vi "ATS_AsyncGetSetBufCount.vi"(9 "Get / Set&Get":bool, 10 "BuffCount":i32, 11 "DeviceIn":i32) -> (0 "Return Code":u32, 2 "BufCount_Out":i32, 3 "DeviceOut":i32)   [LabVIEW 2012]
doc: "_____AlazarTech, Scope_____\n\nGet or Set and Get the Buffer Count use in the AsyncDMA mode.\n\nBuffCount_Out is the value already set for the AsyncDMA read."
uses:
  ATS_ctl/ATS_Global_Ctrl.ctl
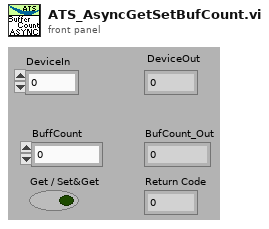
[diagram p1: front panel]
types:
  T1 = typedef "ATS_Global_Ctrl.ctl" = enum16{"Init_Device", "Clear_ALL", "Set", "Get"}
  T2 = typedef "Device_Info.ctl" = cluster{"Handle":u32, "Board":string, "CPLD":string, "MemorySize":u32, "SampleSize":u8, "ID":i32, "High_Memory":bool, "Chan/Board":u8}
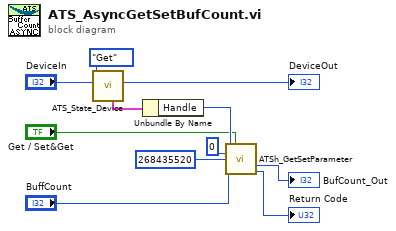
[diagram p0: block diagram]
diagram:
  n1 = call "ATS_State_Device.vi"("DeviceIn"="DeviceIn", "ATS_GBL_Ctrl"=ATS_Global_Ctrl."Get") -> ("DeviceOut"=→"DeviceOut":i32, "DevInfo_Out"=w10:T2)  [unwired: 4 in, 4 out]
  n2 = Unbundle By Name(w10) -> ("Handle"=w8:u32)
  n3 = call "ATSh_GetSetParameter.vi"("Handle"=w8, "Get / Set&Get"="Get / Set&Get", "Channel"=u8 0, "Parameter"=u32 268435520, "Value"="BuffCount") -> ("Value_Out"=→"BufCount_Out":i32, "Return Code"=→"Return Code":u32)  [unwired: 8 in, 1 out]
